vi "CRYGet Default HardwareASIO.vi"(0 "Hardware Cluster In":T1={"Name"="", "Analog I/O"=0, "Digital I/O"=0, "Channels"=2, "Dig Dev ID"=1, "N ports"=3, "Interface"=0, "Dig I/O Ports"=[{"port #"=1, "width"=8, "direction"=0}, {"port #"=2, "width"=8, "direction"=0}, {"port #"=3, "width"=8, "direction"=0}], "Interf settings"=[], "N interfs"=3, "udev SNs"=[], "udev enable"=FALSE, "Channel Array"=[], "Cal sequence"="", "SelectedIn"=0, "SelectedOut"=0, "SelectedTab"=0, "State"=FALSE, "Help"="", "Advanced"=FALSE, "In Audio Driver"=0, "Out Audio Driver"=0} {"Channel Array"."Coupling" items=["Default"=-1, "RSE"=10083, "NRSE"=10078, "Differential"=10106, "Pseudodifferential"=12529]; "Channel Array"."term config" items=["Default"=-1, "RSE"=10083, "NRSE"=10078, "Differential"=10106, "Pseudodifferential"=12529]; "Channel Array"."Anti-aliasing Factor (%fs)" format="%.2f"}) -> (6 "I_Name Out":string[][](array[string]), 8 "O_Name Out":string[][](array[string]), 9 "Hardware Cluster Out":T1={"Name"="", "Analog I/O"=0, "Digital I/O"=0, "Channels"=2, "Dig Dev ID"=1, "N ports"=3, "Interface"=0, "Dig I/O Ports"=[{"port #"=1, "width"=8, "direction"=0}, {"port #"=2, "width"=8, "direction"=0}, {"port #"=3, "width"=8, "direction"=0}], "Interf settings"=[], "N interfs"=3, "udev SNs"=[], "udev enable"=FALSE, "Channel Array"=[], "Cal sequence"="", "SelectedIn"=0, "SelectedOut"=0, "SelectedTab"=0, "State"=FALSE, "Help"="", "Advanced"=FALSE, "In Audio Driver"=0, "Out Audio Driver"=0} {"Channel Array"."Coupling" items=["Default"=-1, "RSE"=10083, "NRSE"=10078, "Differential"=10106, "Pseudodifferential"=12529]; "Channel Array"."term config" items=["Default"=-1, "RSE"=10083, "NRSE"=10078, "Differential"=10106, "Pseudodifferential"=12529]; "Channel Array"."Anti-aliasing Factor (%fs)" format="%.2f"}, 10 "O_Device Info Out":T3(array[cluster]), 11 "AO_Hardware Channel Name Out":string[](array[string]), 12 "I_Device Info Out":T3(array[cluster]), 13 "AI_Hardware Channel Name Out":string[](array[string]), 14 "O_Channel Info Out":T2[](array[typedef]) {"Coupling" items=["Default"=-1, "RSE"=10083, "NRSE"=10078, "Differential"=10106, "Pseudodifferential"=12529]; "term config" items=["Default"=-1, "RSE"=10083, "NRSE"=10078, "Differential"=10106, "Pseudodifferential"=12529]; "Anti-aliasing Factor (%fs)" format="%.2f"}, 15 "I_Channel Info Out":T2[](array[typedef]) {"Coupling" items=["Default"=-1, "RSE"=10083, "NRSE"=10078, "Differential"=10106, "Pseudodifferential"=12529]; "term config" items=["Default"=-1, "RSE"=10083, "NRSE"=10078, "Differential"=10106, "Pseudodifferential"=12529]; "Anti-aliasing Factor (%fs)" format="%.2f"}, 16 "Output Device Name Out":string[](array[string]), 17 "Input Device Name Out":string[](array[string]), 18 "Error":bool, 19 "Device Name Out":string[](array[string]))   [LabVIEW 2013]
uses:
  Typedef Control/CRYHardware Channel Info.ctl
  Typedef Control/CRYHardware.ctl
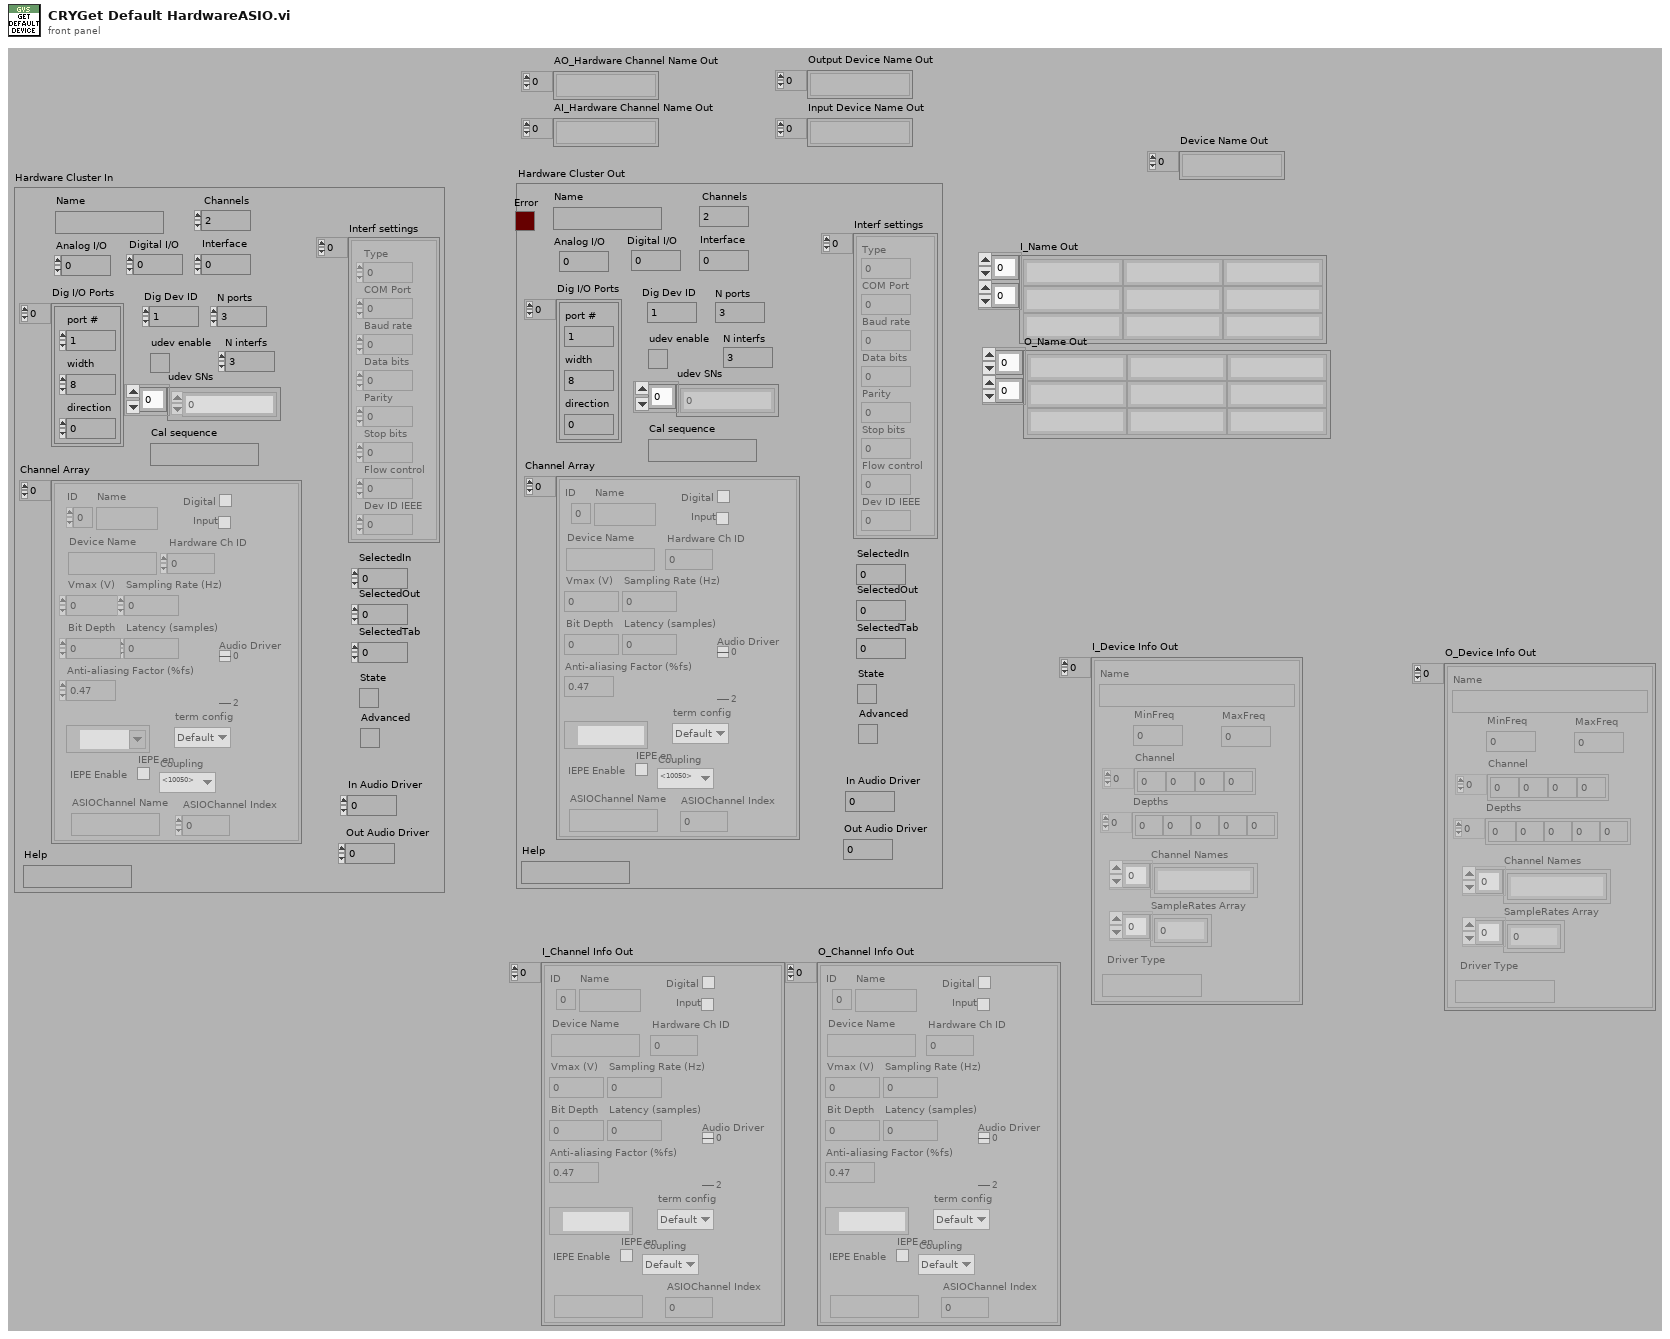
[diagram p1: front panel]
types:
  T1 = typedef "CRYHardware.ctl" = cluster{"Name":string, "Analog I/O":u16, "Digital I/O":u16, "Channels":u8, "Dig Dev ID":u8, "N ports":u8, "Interface":u32, "Dig I/O Ports":cluster{"port #":i16, "width":i16, "direction":i32}[], "Interf settings":cluster{"Type":u16, "COM Port":u8, "Baud rate":u32, "Data bits":u32, "Parity":u16, "Stop bits":u16, "Flow control":u16, "Dev ID IEEE":u8}[], "N interfs":i32, "udev SNs":i16[], "udev enable":bool, "Channel Array":T2[], "Cal sequence":string, "SelectedIn":u16, "SelectedOut":u16, "SelectedTab":u16, "State":bool, "Help":string, "Advanced":bool, "In Audio Driver":u16, "Out Audio Driver":u16}
  T2 = typedef "CRYHardware Channel Info.ctl" = cluster{"ID":i32, "Name":string, "Digital":bool, "Input":bool, "Device Name":string, "Hardware Ch ID":u8, "Vmax (V)":dbl, "Latency (samples)":dbl, "Sampling Rate (Hz)":u32, "Bit Depth":u32, "Anti-aliasing Factor (%fs)":sgl, "DAQmx Channel":tag, "term config":i32, "Coupling":i32, "IEPE en":bool, "ASIOChannel Name":string, "Audio Driver":u16, "ASIOChannel Index":u8}
  T3 = cluster{"Name":string, "MinFreq":dbl, "MaxFreq":dbl, "Channel":i32[], "Depths":i32[], "Channel Names":string[], "SampleRates Array":dbl[], "Driver Type":string}[]
  T4 = cluster{"Type":u16, "COM Port":u8, "Baud rate":u32, "Data bits":u32, "Parity":u16, "Stop bits":u16, "Flow control":u16, "Dev ID IEEE":u8}[]
  T5 = cluster{"port #":i16, "width":i16, "direction":i32}[]
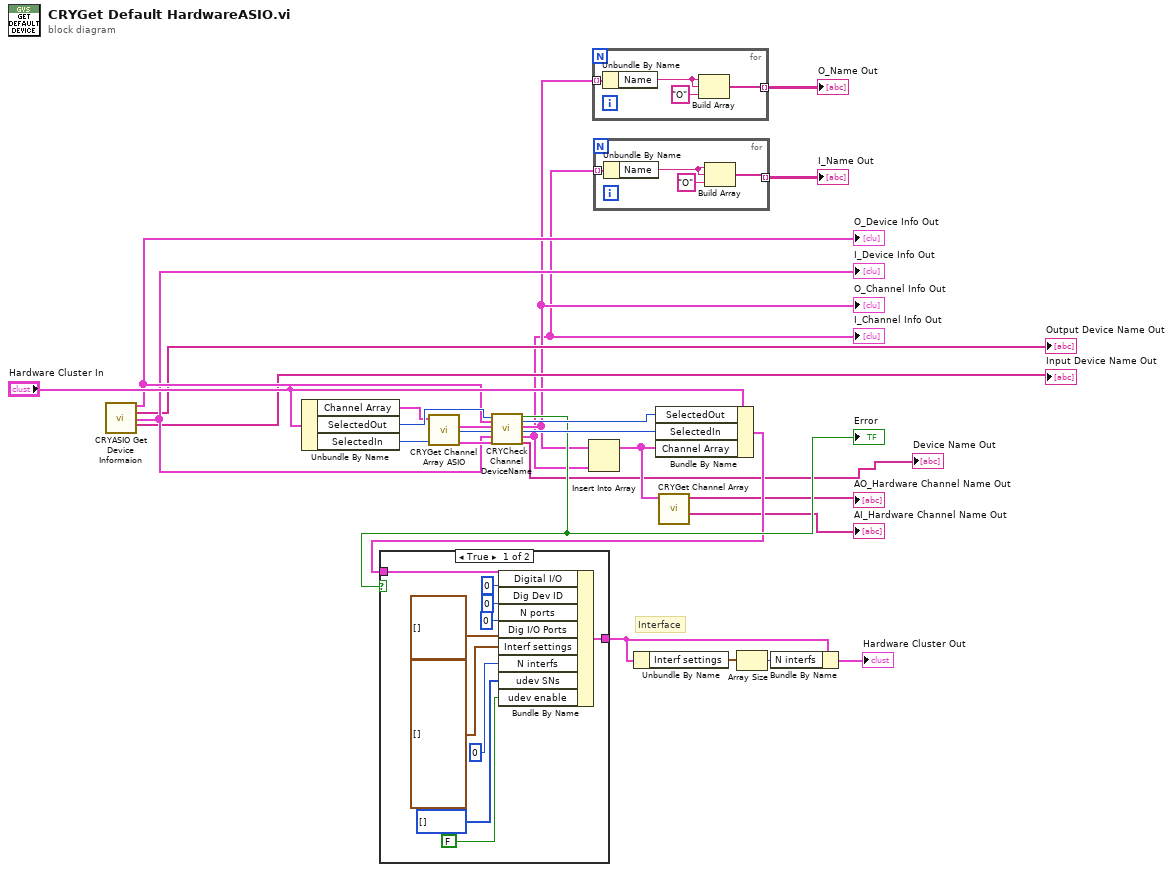
[diagram p0: block diagram]
diagram:
  # "Interface"
  n1 = call "CRYASIO Get Device Informaion.vi"() -> ("ASIO Output Device Infor"=w11:T3, "ASIO Output Device Name"=→"Output Device Name Out":string[], "ASIO Input Device Infor"=w10:T3, "ASIO Input Device Name"=→"Input Device Name Out":string[])  [unwired: 11 in, 1 out]
  "O_Device Info Out" <- w11
  "I_Device Info Out" <- w10
  n2 = Unbundle By Name("Hardware Cluster In") -> ("Channel Array"=w16:T2[], "SelectedOut"=w25:u16, "SelectedIn"=w26:u16)
  n3 = call "CRYGet Channel Array ASIO.vi"("Channel Array"=w16) -> ("I Channel Info Out"=w21:T2[], "O Channel Info Out"=w20:T2[])  [unwired: 7 in, 2 out]
  n4 = call "CRYCheck Channel DeviceName.vi"("SelectedOut"=w25, "O Device Info"=w11, "O Channel Info"=w20, "SelectedIn"=w26, "I Device Info"=w10, "I Channel Info"=w21) -> ("Check State"=w15:bool, "O SelectedN Out"=w22:u16, "O Channel Info Out"=w6:T2[], "I SelectedN Out"=w23:u16, "I Channel Info Out"=w5:T2[], "No Device Name"=→"Device Name Out":string[])  [unwired: 8 out]
  "I_Channel Info Out" <- w5
  "O_Channel Info Out" <- w6
  "Error" <- w15
  n5 = Insert Into Array(array=w6, new element=w5) -> (w24:T2[])  [unwired: 1 in]
  n6 = for {
    tunnel: w6 -> [w30] mode=indexing
    tunnel: [w27] -> w2 mode=indexing
    n7 = Unbundle By Name(w30) -> ("Name"=w29:string)
    n8 = Build Array(w29, w29, "O" ("element")) -> (w27:string[])
  }
  "O_Name Out" <- w2
  n9 = for {
    tunnel: w5 -> [w34] mode=indexing
    tunnel: [w31] -> w3 mode=indexing
    n10 = Unbundle By Name(w34) -> ("Name"=w32:string)
    n11 = Build Array(w32, w32, "O" ("element")) -> (w31:string[])
  }
  "I_Name Out" <- w3
  n12 = Bundle By Name(cluster="Hardware Cluster In", "SelectedOut"=w22, "SelectedIn"=w23, "Channel Array"=w24) -> (w13:T1)
  n13 = case shown="True" w15 {
    tunnel: w13 -> [w44 w45]
    tunnel: [w35 w45] -> w14
    frame True {
      n14 = Bundle By Name(cluster=w44, "Digital I/O"=u16 0, "Dig Dev ID"=u8 0, "N ports"=u8 0, "Dig I/O Ports"=T5 [], "Interf settings"=T4 [], "N interfs"=0, "udev SNs"=i16[] [], "udev enable"=FALSE) -> (w35:T1)
    }
    frame False {
    }
  }
  n15 = Unbundle By Name(w14) -> ("Interf settings"=w17:T4)
  n16 = call "CRYGet Channel Array.vi"("Channel Array"=w24) -> ("I_Channel Name Out"=→"AI_Hardware Channel Name Out":string[], "O_Channel Name Out"=→"AO_Hardware Channel Name Out":string[])  [unwired: 9 out]
  n17 = Array Size(array=w17) -> (size(s)=w18:i32)
  n18 = Bundle By Name(cluster=w14, "N interfs"=w18) -> (→"Hardware Cluster Out":T1)
